vi "svl_Check Data Valid [Integration] (N Ch).vi"(0 "scaled signals [EU]":waveform(dbl)[](array[waveform]), 1 "reset (in)":bool, 5 "integration type":T1(ring)=enum."double integration", 7 "highpass cutoff frequency":dbl=1.0 format="%.2f", 11 "error in (no error)":errorcluster) -> (3 "reset (out)":bool, 4 "integrated signals":waveform(dbl)[](array[waveform]), 6 "dup integration type":T1(ring)=enum."double integration", 8 "dup highpass cutoff frequency":dbl=1.0 format="%.2f", 15 "error out":errorcluster)   [LabVIEW 2017, in "SoundVib_Integration.lvlib"]
uses:
  <vilib>/addons/Sound and Vibration/svt_Integration/SoundVib_Integration.lvlib
  <vilib>/addons/_NISVFA/_Shared subVIs/Common/svc_Check for Waveform Parameter Continuity (no state).vi
  <vilib>/addons/_NISVFA/_Shared subVIs/Common/svc_Get SV Channel Info.vi
  <vilib>/addons/_NISVFA/_Shared subVIs/Common/svc_Engineering Units to Unit Label.vi
  <vilib>/addons/_NISVFA/_Shared subVIs/Common/svc_Unit Label to Engineering Units.vi
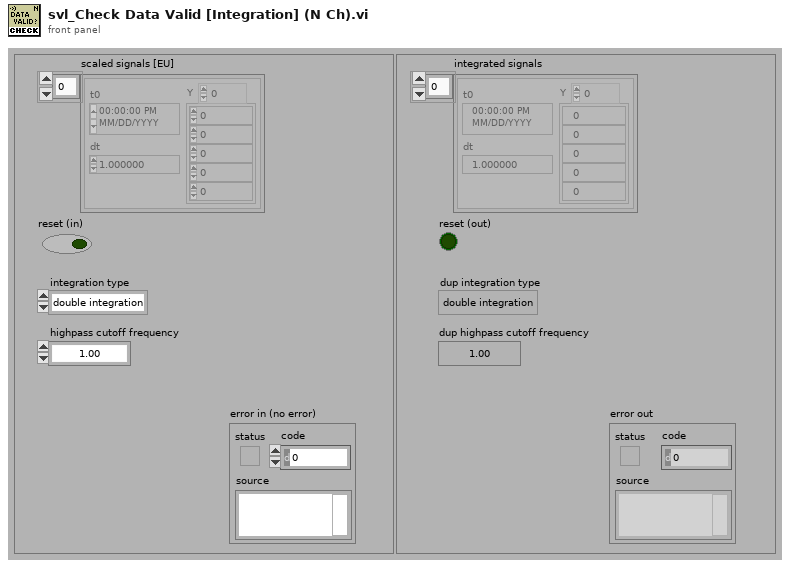
[diagram p1: front panel]
types:
  T1 = enum16{"single integration", "double integration"}
  T2 = cluster{"dt equal":bool, "array length equal":bool, "number channels change":bool}
  T3 = cluster{"dt":bool, "t0 continuity":bool, "array length":bool, "channel info":bool, "name":bool}
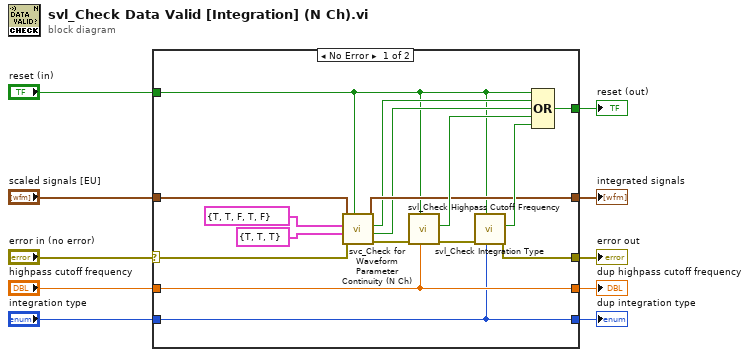
[diagram p0: block diagram]
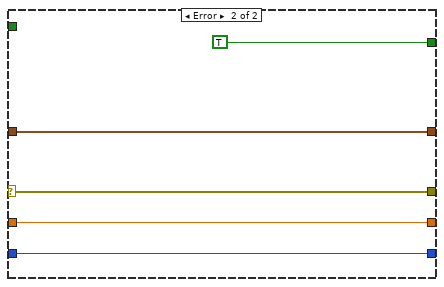
[diagram p2: hidden frame]
diagram:
  n1 = case shown="No Error" "error in (no error)" {
    selector: "error in (no error)" -> [w19 w31]
    tunnel: "scaled signals [EU]" -> [w17 w27]
    tunnel: [w26 TRUE ("t0 changed")] -> w8
    tunnel: [w24 w31] -> w7
    tunnel: [w16 w27] -> w1
    tunnel: "reset (in)" -> [w13 _]
    tunnel: "highpass cutoff frequency" -> [w21 w29]
    tunnel: "integration type" -> [w20 w28]
    tunnel: [w21 w29] -> w3
    tunnel: [w20 w28] -> w2
    frame No Error {
      n2 = call <vilib>:"svc_Check for Waveform Parameter Continuity (N Ch).vi"("restart averaging (F)"=w13, "error in (no error)"=w19, "checks for multichannel parameters"=T2 {"dt equal"=TRUE, "array length equal"=TRUE, "number channels change"=TRUE}, "checks for channel parameter change"=T3 {"dt"=TRUE, "t0 continuity"=TRUE, "array length"=FALSE, "channel info"=TRUE, "name"=FALSE}, "scaled signal(s)"=w17) -> ("error out"=w18:errorcluster, "multichannel parameter changed"=w14:bool, "waveform parameter changed"=w15:bool, "dup scaled signal(s)"=w16:waveform(dbl)[])  [unwired: 3 out]
      n3 = call <vilib>:"svl_Check Highpass Cutoff Frequency.vi"("highpass cutoff frequency"=w21, "reset (in)"=w13, "error in (no error)"=w18) -> ("error out"=w25:errorcluster, "parameter has changed"=w23:bool)  [unwired: 7 in]
      n4 = call <vilib>:"svl_Check Integration Type.vi"("integration type"=w20, "reset (in)"=w13, "error in (no error)"=w25) -> ("error out"=w24:errorcluster, "parameter has changed"=w22:bool)  [unwired: 7 in]
      n5 = Compound Arithmetic op=OR(w13, w15, w14, w23, w22) -> (w26:bool)
    }
    frame Error {
    }
  }
  "error out" <- w7
  "integrated signals" <- w1
  "reset (out)" <- w8
  "dup integration type" <- w2
  "dup highpass cutoff frequency" <- w3
